vi "PH_Powermeter_BaseClass.set i Attr and open DIM services.vi"(0 "i ref in":refnum<vi>, 5 "error in":errorcluster) -> (14 "i ref out":refnum<vi>, 16 "i Attributes":T1={"GUI References"={"Head Attributes"=refnum, "Energy"=refnum, "Connection"=refnum, "VISA Resource"=refnum, "Energy evolution"=refnum, "Scaling Factor"=refnum, "Range"=refnum, "Wavelength"=refnum, "Trigger Level"=refnum, "Wanted Settings"=refnum, "Current Settings"=refnum}, "Connection"={"failed checks"=0, "Timeout"=FALSE, "Data read"="", "Failure"=FALSE, "Error"=FALSE, "State"=enum."off"}, "Head Attributes"={"Instrument Type"="", "Head Version"="", "Head Name"="", "Serial Number"="", "Firmware"="", "Sensor Type"="---", "MinimumRange"=0, "Maximum Range"=0, "Min Wavelength"=0, "Max Wavelength"=0}, "VISA resource"="", "Energy"={"current Value"=0.0, "unscaled"=0.0, "Scaling Factor"=0.0}, "Service ID Energy"=-1, "Wanted Settings"={"Trigger Level"=0.0, "Wavelength"=1, "Range"=0}, "Current Settings"={"Trigger Level"=0.0, "Wavelength"=1, "Range"=0}} {"Energy"."unscaled" format="%#_6p"; "Energy"."current Value" format="%#.1p"}, 19 "error out":errorcluster)   [LabVIEW 2014, in "PH_Powermeter_BaseClass.lvlib"]
doc: "This VI reads the DB entries and sets several attributes and GUI element settings."
uses:
  PH_Powermeter_BaseClass.lvlib
  PH_Powermeter_BaseClass.i attribute.ctl
  PH_Powermeter_BaseClass.GUI Refs.ctl
  PH_Powermeter_BaseClass.Head Attributes.ctl
  PH_Powermeter_BaseClass.Energy.ctl
  PH_Powermeter_BaseClass.Connection.ctl
  PH_Powermeter_BaseClass.State.ctl
  PH_gentec_BaseClass.Head Settings.ctl
  PH_Common/PH_Common.lvlib
  CS_Core/CSSystem/CSSystemLib/CSSystemLib.lvlib
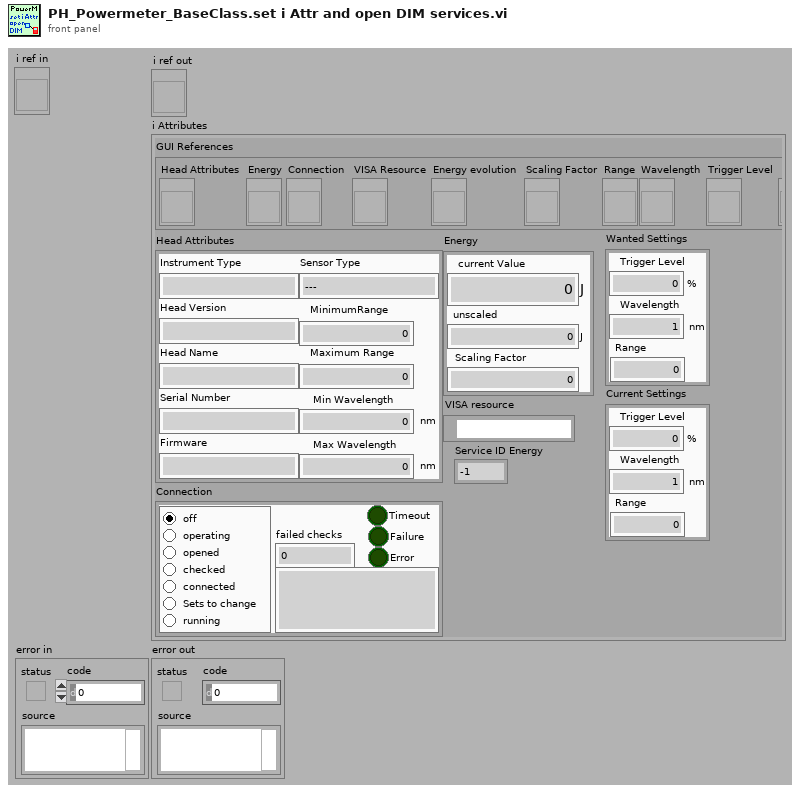
[diagram p1: front panel]
types:
  T1 = typedef "PH_Powermeter_BaseClass.lvlib/PH_Powermeter_BaseClass.i attribute.ctl" = cluster{"GUI References":T2, "Connection":T3, "Head Attributes":T5, "VISA resource":refnum<visa-resource-name>, "Energy":T6, "Service ID Energy":i32, "Wanted Settings":T7, "Current Settings":T7}
  T2 = typedef "PH_Powermeter_BaseClass.lvlib/PH_Powermeter_BaseClass.GUI Refs.ctl" = cluster{"Head Attributes":refnum<vi>, "Energy":refnum<vi>, "Connection":refnum<vi>, "VISA Resource":refnum<vi>, "Energy evolution":refnum<vi>, "Scaling Factor":refnum<vi>, "Range":refnum<vi>, "Wavelength":refnum<vi>, "Trigger Level":refnum<vi>, "Wanted Settings":refnum<vi>, "Current Settings":refnum<vi>}
  T3 = typedef "PH_Powermeter_BaseClass.lvlib/PH_Powermeter_BaseClass.Connection.ctl" = cluster{"failed checks":i8, "Timeout":bool, "Data read":string, "Failure":bool, "Error":bool, "State":T4}
  T4 = typedef "PH_Powermeter_BaseClass.lvlib/PH_Powermeter_BaseClass.State.ctl" = enum32{"off", "operating", "opened", "checked", "connected", "Sets to change", "running"}
  T5 = typedef "PH_Powermeter_BaseClass.lvlib/PH_Powermeter_BaseClass.Head Attributes.ctl" = cluster{"Instrument Type":string, "Head Version":string, "Head Name":string, "Serial Number":string, "Firmware":string, "Sensor Type":string, "MinimumRange":u32, "Maximum Range":u32, "Min Wavelength":i32, "Max Wavelength":i32}
  T6 = typedef "PH_Powermeter_BaseClass.lvlib/PH_Powermeter_BaseClass.Energy.ctl" = cluster{"current Value":dbl, "unscaled":dbl, "Scaling Factor":dbl}
  T7 = typedef "PH_Powermeter_BaseClass.lvlib/PH_gentec_BaseClass.Head Settings.ctl" = cluster{"Trigger Level":dbl, "Wavelength":u32, "Range":u32}
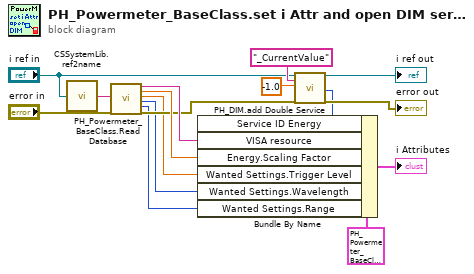
[diagram p0: block diagram]
diagram:
  n1 = call "CSSystemLib.ref2name.vi"("obj refnum"="i ref in") -> ("name"=w11:string)
  n2 = call "PH_Powermeter_BaseClass.Read Database.vi"("Instance Name"=w11, "error in"="error in") -> ("VISA Resource"=w13:string, "Scaling Factor"=w14:dbl, "Trigger Level [%]"=w3:dbl, "Wavelength [nm]"=w2:u32, "Range"=w1:u32, "error out"=w8:errorcluster)  [unwired: 12 in]
  n3 = call "PH_DIM.add Double Service.vi"("i ref in"="i ref in", "Service Name"="_CurrentValue", "Double Value"=-1.0, "error in (no error)"=w8) -> ("i ref out"=→"i ref out":refnum<vi>, "Service ID"=w4:i32, "error out"=→"error out":errorcluster)  [unwired: 13 in]
  n4 = Bundle By Name(cluster=T1 {"GUI References"={"Head Attributes"=refnum, "Energy"=refnum, "Connection"=refnum, "VISA Resource"=refnum, "Energy evolution"=refnum, "Scaling Factor"=refnum, "Range"=refnum, "Wavelength"=refnum, "Trigger Level"=refnum, "Wanted Settings"=refnum, "Current Settings"=refnum}, "Connection"={"failed checks"=0, "Timeout"=FALSE, "Data read"="", "Failure"=FALSE, "Error"=FALSE, "State"=enum."off"}, "Head Attributes"={"Instrument Type"="", "Head Version"="", "Head Name"="", "Serial Number"="", "Firmware"="", "Sensor Type"="---", "MinimumRange"=0, "Maximum Range"=0, "Min Wavelength"=0, "Max Wavelength"=0}, "VISA resource"="", "Energy"={"current Value"=0.0, "unscaled"=0.0, "Scaling Factor"=0.0}, "Service ID Energy"=-1, "Wanted Settings"={"Trigger Level"=0.0, "Wavelength"=1, "Range"=0}, "Current Settings"={"Trigger Level"=0.0, "Wavelength"=1, "Range"=0}} ("CLASS.i attribute"), "Service ID Energy"=w4, "VISA resource"=w13, "Energy.Scaling Factor"=w14, "Wanted Settings.Trigger Level"=w3, "Wanted Settings.Wavelength"=w2, "Wanted Settings.Range"=w1) -> (→"i Attributes":T1)
